vi "CSM - Wait for Module to Be Alive.vi"(0 "Target Module":string, 9 "Wait(5000ms)":i32=5000, 11 "error in (no error)":errorcluster) -> (4 "Target Module (dup)":string, 10 "Waited(ms)":u32, 15 "error out":errorcluster)   [LabVIEW 2020, in "Communicable State Machine.lvlib"]
uses:
  Communicable State Machine.lvlib
  Priority Queue.lvclass/Priority Queue.ctl
  _Obtain CSM Data Queue.vi
  Release Priority Queue.vi
  Obtain Priority Queue.vi
  CSM No Target Error.vi
  Priority Queue.lvclass
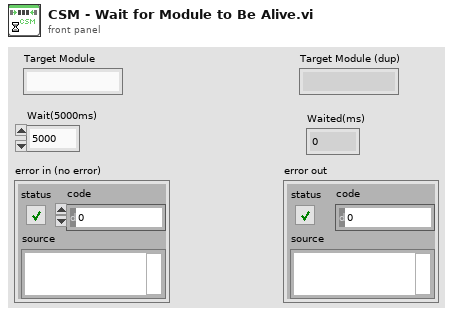
[diagram p1: front panel]
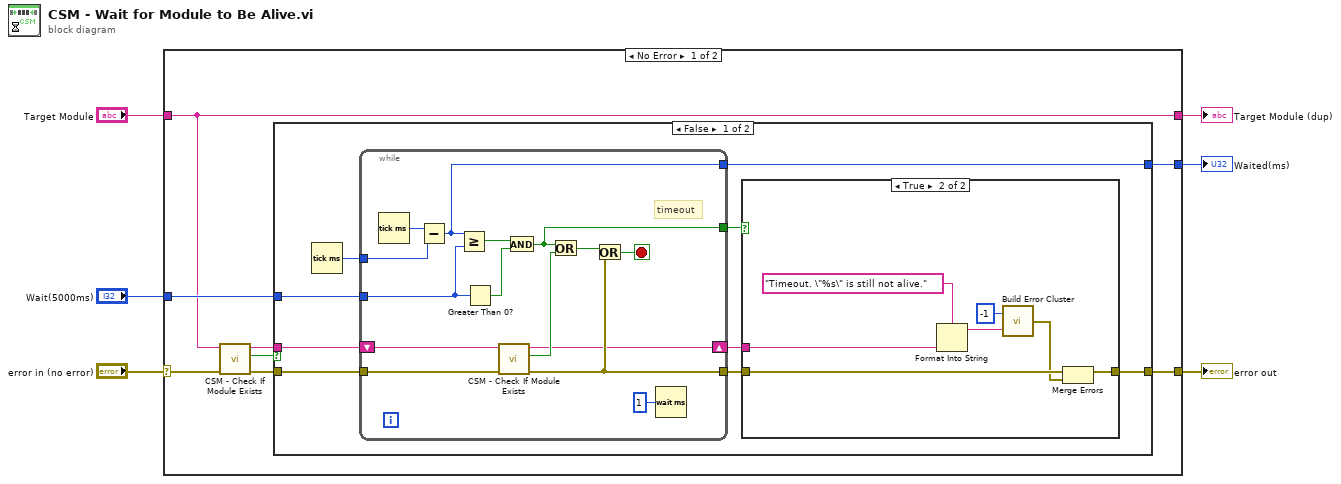
[diagram p0: block diagram]
diagram:
  n1 = case shown="No Error" "error in (no error)" {
    selector: "error in (no error)" -> [w12 w49]
    tunnel: [w14 w49] -> w6
    tunnel: "Wait(5000ms)" -> [w13 _]
    tunnel: "Target Module" -> [w10 w48]
    tunnel: [w10 w48] -> w2
    tunnel: [w7 _] -> w1
    frame No Error {
      n2 = call "CSM - Check If Module Exists.vi"("Error in"=w12, "CSM Name"=w10) -> ("Error out"=w11:errorcluster, "Exist?"=w8:bool, "CSM Name(dup)"=w9:string)  [unwired: 7 in]
      n3 = case shown="False" w8 {
        tunnel: [w21 w47] -> w14
        tunnel: w13 -> [w19 _]
        tunnel: w11 -> [w17 w47]
        tunnel: w9 -> [w16 _]
        tunnel: [w15 _] -> w7
        frame False {
          n4 = Tick Count (ms)() -> (millisecond timer value=w18:u32)
          n5 = while {
            tunnel: w18 -> [w45]
            tunnel: w19 -> [w43]
            tunnel: w17 -> [w40]
            tunnel: [w36] -> w22
            tunnel: [w35] -> w20
            shift-right: [w34] -> w23
            shift-left: w16 -> [w41]
            tunnel: [w32] -> w15
            stop <- w38 stop-if-true
            # "timeout"
            n6 = Tick Count (ms)() -> (millisecond timer value=w46:u32)
            n7 = Subtract(x=w46, y=w45) -> (x-y=w32:u32)
            n8 = Greater Or Equal?(x=w32, y=w43) -> (x >= y?=w44:bool)
            n9 = Greater Than 0?(x=w43) -> (x > 0?=w42:bool)
            n10 = call "CSM - Check If Module Exists.vi"("Error in"=w40, "CSM Name"=w41) -> ("Error out"=w36:errorcluster, "Exist?"=w39:bool, "CSM Name(dup)"=w34:string)  [unwired: 7 in]
            n11 = And(x=w44, y=w42) -> (x .and. y?=w35:bool)
            n12 = Or(x=w35, y=w39) -> (x .or. y?=w37:bool)
            n13 = Or(x=w37, y=w36) -> (x .or. y?=w38:bool)
            n14 = Wait (ms)(milliseconds to wait=u32 1) -> ()  [unwired: 1 out]
          }
          n15 = case shown="True" w20 {
            tunnel: [w24 w30] -> w21
            tunnel: w22 -> [w24 w31]
            tunnel: w23 -> [_ w25]
            frame False {
            }
            frame True {
              n16 = Format Into String(format string="Timeout. \"%s\" is still not alive.", w25) -> (resulting string=w27:string)  [unwired: 2 in, 1 out]
              n17 = call "Build Error Cluster.vi"("String to Prepend to source (\"\")"=w27, "code"=-1) -> ("error out"=w29:errorcluster)
              n18 = Merge Errors(w31, w29) -> (w30:errorcluster)
            }
          }
        }
        frame True {
        }
      }
    }
    frame Error {
    }
  }
  "error out" <- w6
  "Target Module (dup)" <- w2
  "Waited(ms)" <- w1
